vi "P偏移矩形（TB）.vi"(10 "RectTB":T1, 11 "point":cluster{"x":i16, "y":i16} caption="点") -> (3 "RectTB(Offset)":T1)   [LabVIEW 2011]
uses:
  RectTB.ctl
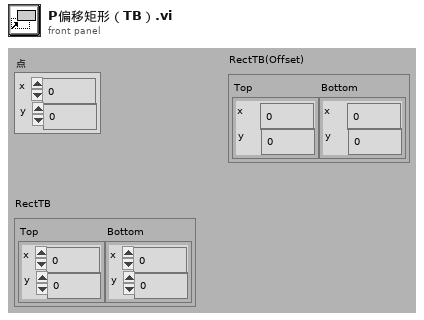
[diagram p1: front panel]
types:
  T1 = typedef "RectTB.ctl" = cluster{"Top":cluster{"x":i16, "y":i16}, "Bottom":cluster{"x":i16, "y":i16}}
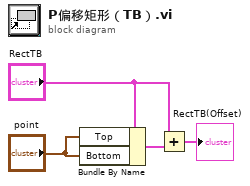
[diagram p0: block diagram]
diagram:
  n1 = Bundle By Name(cluster="RectTB", "Top"="point", "Bottom"="point") -> (w3:T1)
  n2 = Add(x="RectTB", y=w3) -> (x+y=→"RectTB(Offset)":T1)
